vi "Write input_.vi"(8 "error in":errorcluster, 10 "input?":bool, 11 "decideprojectfeatures in":refnum<class "DecideModuleFeatures.lvclass">) -> (0 "error out":errorcluster, 3 "decideprojectfeatures out":refnum<class "DecideModuleFeatures.lvclass">)   [LabVIEW 2013, in "DecideModuleFeatures.lvclass"]
uses:
  DecideModuleFeatures.lvclass
  DecideModuleFeatures.lvclass/DecideModuleFeatures.ctl
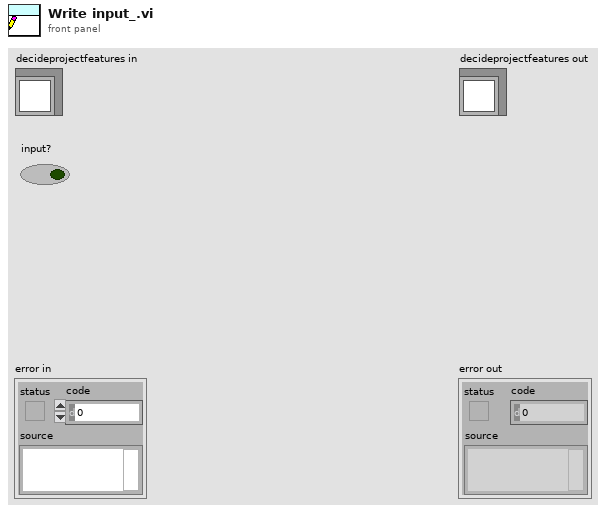
[diagram p1: front panel]
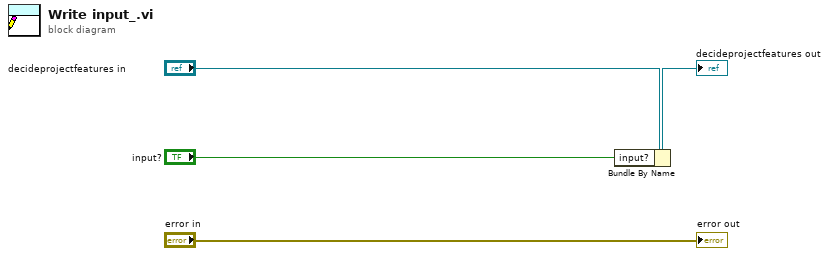
[diagram p0: block diagram]
diagram:
  n1 = Bundle By Name(cluster="decideprojectfeatures in", "input?"="input?") -> (→"decideprojectfeatures out":refnum<class "DecideModuleFeatures.lvclass">)
  "error out" <- "error in"
